vi "Test_Reactor Temperature Rise Redundancy.vi"() -> ()   [LabVIEW 2022 SP3]
uses:
  SI_modules/SI100/SI100.lvclass
panel:
  out "Avg Temp rise":cluster{"Time":timestamp[], dbl[]}(graph)
  out "Inputs":cluster{"Time":timestamp[], dbl[]}[](graph)
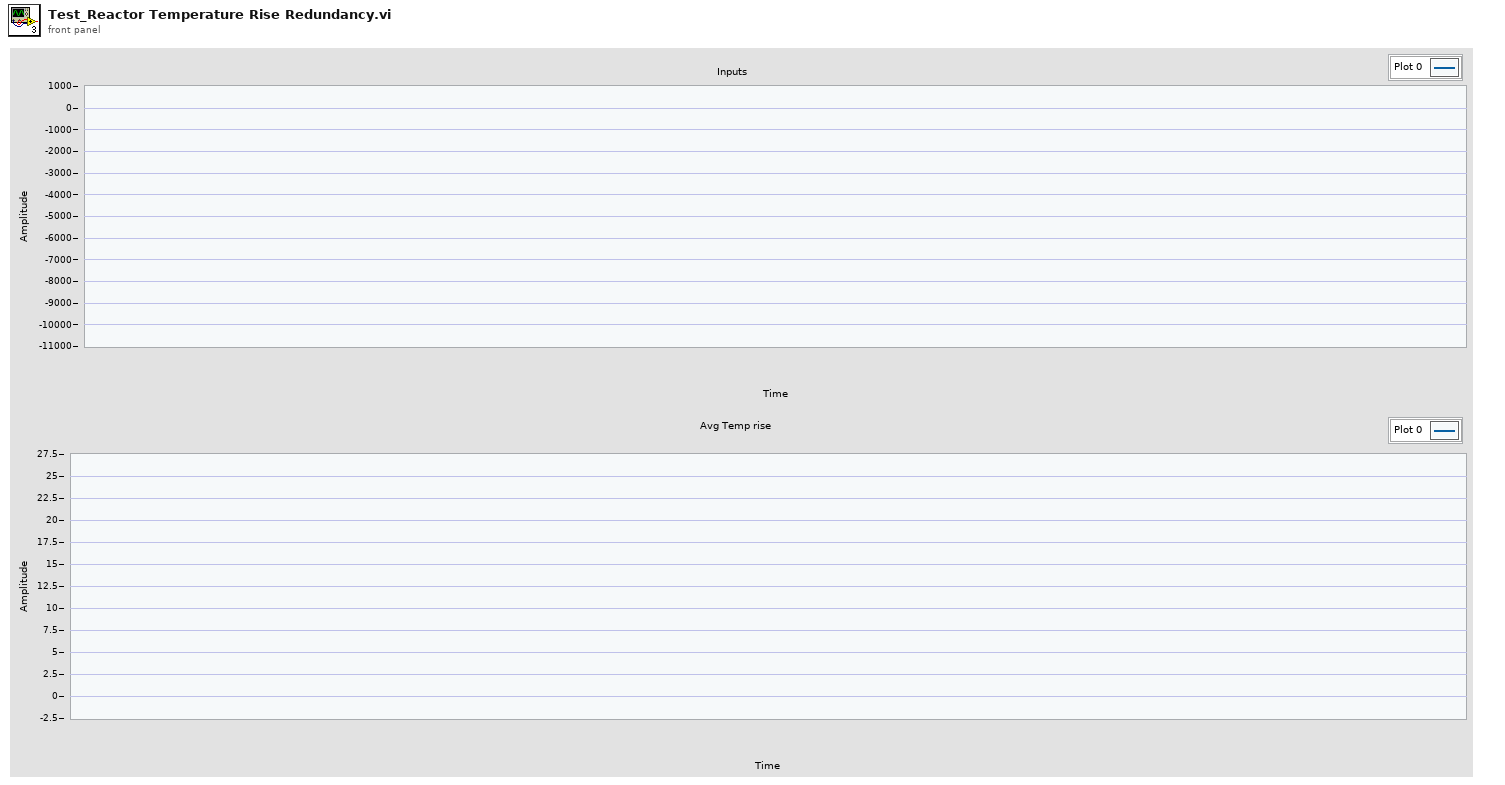
[diagram p1: front panel]
types:
  T1 = cluster{"[0]":cluster{"Time":timestamp[], "KKS":string, "Meas":dbl[]}, "[1]":cluster{"Time":timestamp[], "KKS":string, "Meas":dbl[]}, "[2]":cluster{"Time":timestamp[], "KKS":string, "Meas":dbl[]}, "[3]":cluster{"Time":timestamp[], "KKS":string, "Meas":dbl[]}, "[4]":cluster{"Time":timestamp[], "KKS":string, "Meas":dbl[]}, "[5]":cluster{"Time":timestamp[], "KKS":string, "Meas":dbl[]}, "[6]":cluster{"Time":timestamp[], "KKS":string, "Meas":dbl[]}, "[7]":cluster{"Time":timestamp[], "KKS":string, "Meas":dbl[]}, "[8]":cluster{"Time":timestamp[], "KKS":string, "Meas":dbl[]}}
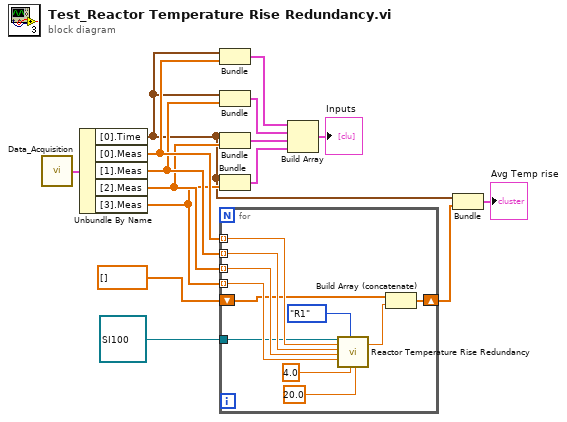
[diagram p0: block diagram]
diagram:
  n1 = call "Data_Acquisition.vi"() -> ("Meas"=w15:T1)  [unwired: 15 in]
  n2 = Unbundle By Name(w15) -> ("[0].Time"=w2:timestamp[], "[0].Meas"=w14:dbl[], "[1].Meas"=w13:dbl[], "[2].Meas"=w12:dbl[], "[3].Meas"=w11:dbl[])
  n3 = Bundle("Time"=w2, "Meas"=w14) -> (w10:cluster{"Time":timestamp[], "Meas":dbl[]})  [unwired: 1 in]
  n4 = Bundle("Time"=w2, "Meas"=w13) -> (w9:cluster{"Time":timestamp[], "Meas":dbl[]})  [unwired: 1 in]
  n5 = Bundle("Time"=w2, "Meas"=w12) -> (w8:cluster{"Time":timestamp[], "Meas":dbl[]})  [unwired: 1 in]
  n6 = Bundle("Time"=w2, "Meas"=w11) -> (w7:cluster{"Time":timestamp[], "Meas":dbl[]})  [unwired: 1 in]
  n7 = for {
    tunnel: refnum<class "SI100.lvclass"> refnum ("SI100.lvclass") -> [w20]
    tunnel: w14 -> [w24] mode=indexing
    tunnel: w13 -> [w23] mode=indexing
    tunnel: w12 -> [w22] mode=indexing
    tunnel: w11 -> [w21] mode=indexing
    shift-right: [w18] -> w4
    shift-left: dbl[] [] -> [w16]
    n8 = call "Reactor Temperature Rise Redundancy.vi"("SI100_ReactorTemperatureRise.lvclass"=w20, "3 JEC CT951 XQ01"=w24, "3 JEC CT952 XQ01"=w23, "3 JEC CT953 XQ01"=w22, "3 JEC CT954 XQ01"=w21, "Redundancy"=enum16{"R1", "R2", "R3", "R4"}."R1", "In1"=4.0, "In2"=20.0) -> ("Avg Temp Rise"=w17:dbl)  [unwired: 8 in, 3 out]
    n9 = Build Array (concatenate)(w16, w17) -> (w18:dbl[])
  }
  n10 = Build Array(w10, w9, w8, w7) -> (→"Inputs":cluster{"Time":timestamp[], "Meas":dbl[]}[])
  n11 = Bundle("Time"=w2, w4) -> (→"Avg Temp rise":cluster{"Time":timestamp[], dbl[]})  [unwired: 1 in]
